vi "__RunTestsInCurrentProject.vi"() -> ()   [LabVIEW 2019]
uses:
  TestResult/TestResult.lvclass
  TestRunner/TestRunner.lvclass
  <vilib>/Analysis/baseanly.llb/Mean (DBL).vi
  TestSuite/TestSuite.lvclass
  TestFailure/TestFailure.lvclass
  CodeCoverage/CodeCoverage.lvclass
  <vilib>/Analysis/NI_AALBase.lvlib
panel:
  out "Not Fully Covered":path[](array[path])
  out "Total Coverage [%]":dbl format="%0.2f"
  out "Time [s]":dbl
  out "Count":i32
  out "error out":errorcluster
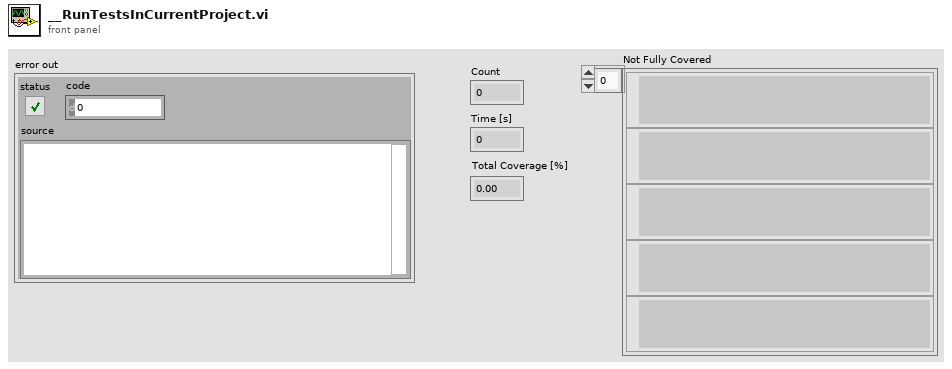
[diagram p1: front panel]
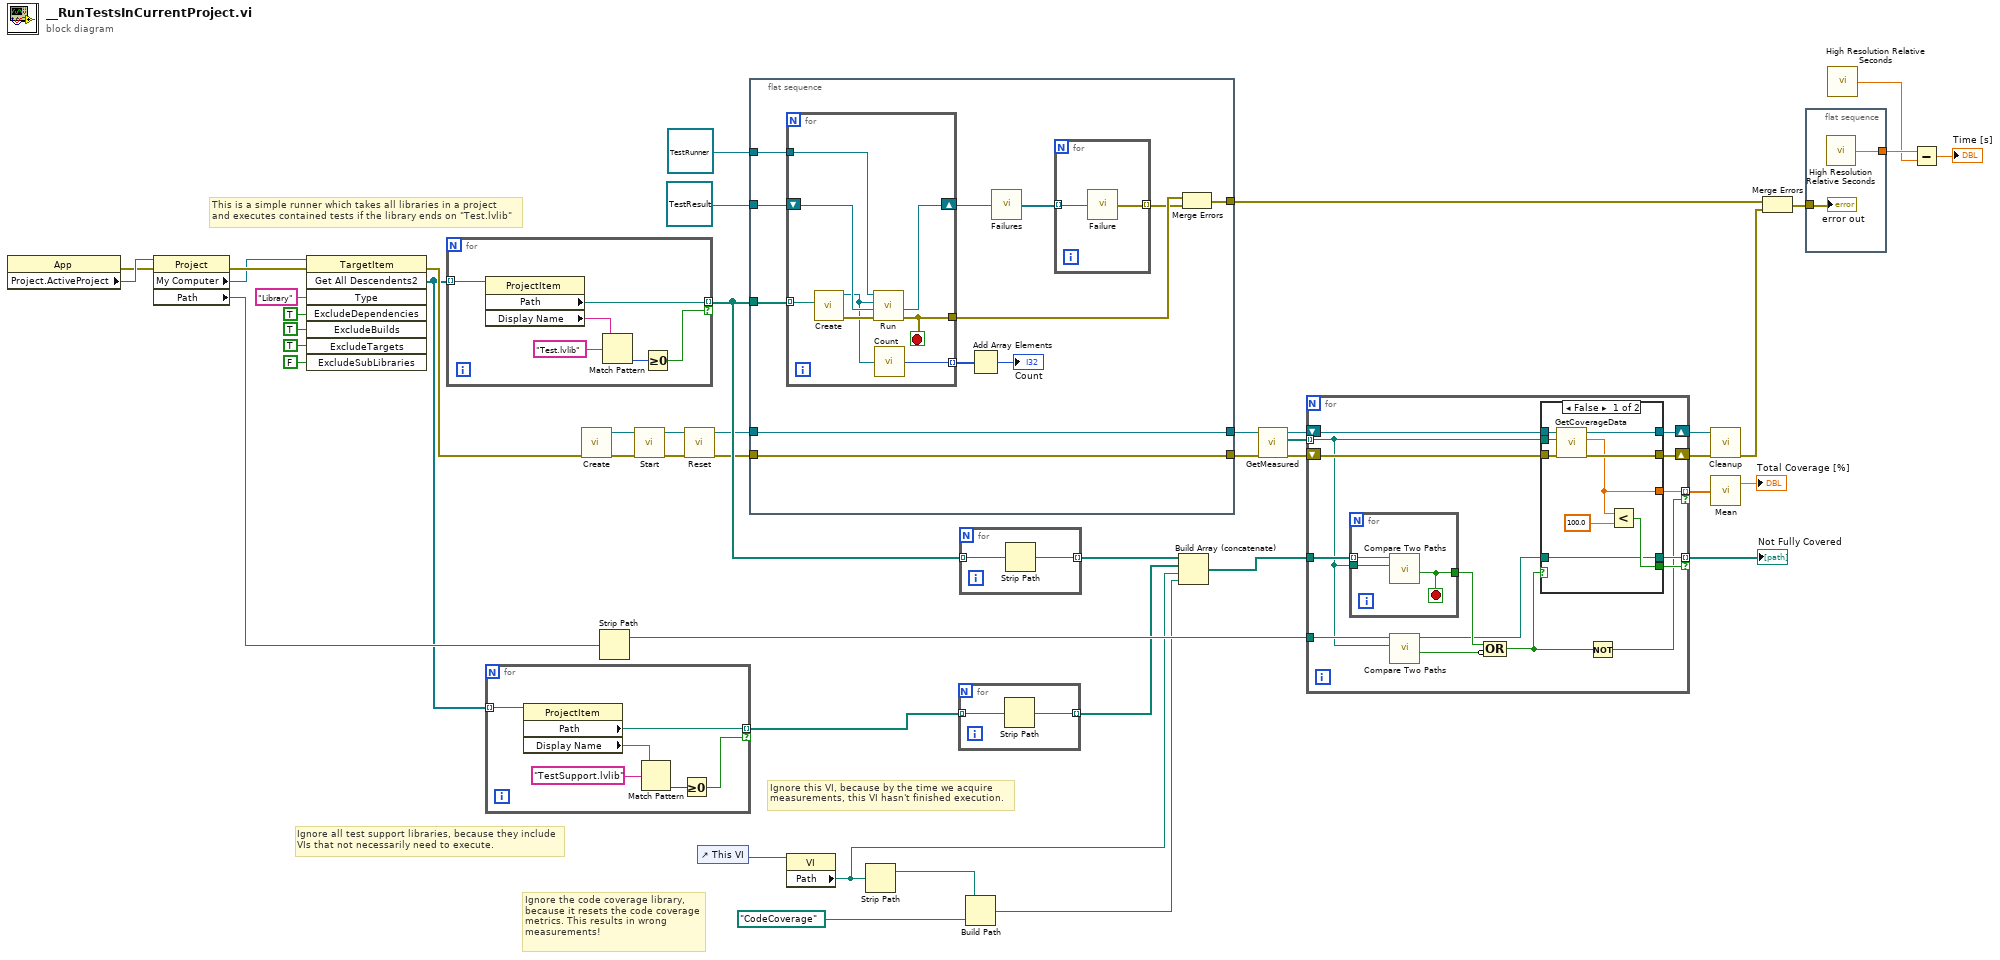
[diagram p0: block diagram]
diagram:
  # "Ignore all test support libraries, because they include\nVIs that not necessarily need to execute."
  # "Ignore this VI, because by the time we acquire\nmeasurements, this VI hasn't finished execution."
  # "Ignore the code coverage library,\nbecause it resets the code coverage\nmetrics. This results in wrong\nmeasurements!"
  # "This is a simple runner which takes all libraries in a project\nand executes contained tests if the library ends on \"Test.lvlib\""
  n1 = property class="App"() -> (error out=w46:errorcluster, "Project.ActiveProject"=w47:refnum<vi>)  [unwired: 2 in, 1 out]
  n2 = property class="Project"(reference=w47, error in=w46) -> (error out=w45:errorcluster, "My Computer"=w34:refnum<vi>, "Path"=w18:path)  [unwired: 1 out]
  n3 = invoke class="TargetItem" method="Get All Descendents2"(reference=w34, error in=w45, "Type"="Library", "ExcludeDependencies"=TRUE, "ExcludeBuilds"=TRUE, "ExcludeTargets"=TRUE, "ExcludeSubLibraries"=FALSE) -> (error out=w20:errorcluster, "Get All Descendents2"=w14:refnum<vi>[])  [unwired: 1 in, 6 out]
  n4 = for {
    tunnel: w14 -> [w53] mode=indexing
    tunnel: [w49] -> w17 mode=indexing if=w48
    n5 = property class="ProjectItem"(reference=w53) -> ("Path"=w49:path, "Display Name"=w50:string)  [unwired: 1 in, 2 out]
    n6 = Match Pattern(string=w50, regular expression="Test.lvlib") -> (offset past match=w51:i32)  [unwired: 1 in, 3 out]
    n7 = Greater Or Equal To 0?(x=w51) -> (x >= 0?=w48:bool)
  }
  n8 = for {
    tunnel: w14 -> [w59] mode=indexing
    tunnel: [w55] -> w13 mode=indexing if=w54
    n9 = property class="ProjectItem"(reference=w59) -> ("Path"=w55:path, "Display Name"=w56:string)  [unwired: 1 in, 2 out]
    n10 = Match Pattern(string=w56, regular expression="TestSupport.lvlib") -> (offset past match=w57:i32)  [unwired: 1 in, 3 out]
    n11 = Greater Or Equal To 0?(x=w57) -> (x >= 0?=w54:bool)
  }
  n12 = call "Create.vi"("error in (no error)"=w20) -> ("error out"=w31:errorcluster, "CodeCoverage out"=w4:refnum<class "CodeCoverage.lvclass">)  [unwired: 9 in]
  n13 = Strip Path(path=w18) -> (stripped path=w15:path)  [unwired: 1 out]
  n14 = call "Start.vi"("error in (no error)"=w31, "CodeCoverage in"=w4) -> ("error out"=w6:errorcluster, "CodeCoverage out"=w3:refnum<class "CodeCoverage.lvclass">)  [unwired: 8 in]
  n15 = call "Reset.vi"("error in (no error)"=w6, "CodeCoverage in"=w3) -> ("error out"=w5:errorcluster, "CodeCoverage out"=w2:refnum<class "CodeCoverage.lvclass">)  [unwired: 8 in]
  n16 = control-ref of="This VI"() -> (w10:refnum<vi>)
  n17 = flat-sequence {
    tunnel: w17 -> [w71]
    tunnel: refnum<class "TestResult.lvclass"> refnum ("TestResult out") -> [w70]
    tunnel: [w65] -> w29
    tunnel: refnum<class "TestRunner.lvclass"> refnum ("TestRunner in") -> [w64]
    tunnel: [w61] -> w23
    tunnel: w2 -> [w61]
    tunnel: [w60] -> w32
    tunnel: w5 -> [w60]
    frame #0 {
      n18 = for {
        tunnel: w71 -> [w81] mode=indexing
        shift-right: [w79] -> w69
        shift-left: w70 -> [w80]
        tunnel: [w77] -> w67
        tunnel: w64 -> [w76]
        tunnel: [w74] -> w63 mode=indexing
        stop <- w77 stop-if-true
        n19 = call "Create.vi"("Path"=w81) -> ("error out"=w78:errorcluster, "TestSuite"=w75:refnum<class "TestSuite.lvclass">)  [unwired: 9 in]
        n20 = call-dynamic "Run.vi"("error in (no error)"=w78, "TestResult"=w80, "TestSuite"=w75, "TestRunner in"=w76) -> ("error out"=w77:errorcluster, "TestResult out"=w79:refnum<class "TestResult.lvclass">)  [unwired: 5 in, 1 out]
        n21 = call "Count.vi"("TestSuite In"=w75) -> ("Count"=w74:i32)
      }
      n22 = Add Array Elements(numeric array=w63) -> (sum=→"Count":i32)
      n23 = call "Failures.vi"("TestResult In"=w69) -> ("Failures"=w68:refnum<class "TestFailure.lvclass">[])
      n24 = for {
        tunnel: w68 -> [w73] mode=indexing
        tunnel: [w72] -> w66 mode=indexing
        n25 = call "Failure.vi"("TestFailure In"=w73) -> ("Failure"=w72:errorcluster)
      }
      n26 = Merge Errors(w67, w66) -> (w65:errorcluster)
    }
  }
  n27 = property class="VI"(reference=w10) -> ("Path"=w7:path)  [unwired: 1 in, 2 out]
  n28 = Strip Path(path=w7) -> (stripped path=w8:path)  [unwired: 1 out]
  n29 = for {
    tunnel: w13 -> [w83] mode=indexing
    tunnel: [w82] -> w11 mode=indexing
    n30 = Strip Path(path=w83) -> (stripped path=w82:path)  [unwired: 1 out]
  }
  n31 = for {
    tunnel: w17 -> [w85] mode=indexing
    tunnel: [w84] -> w16 mode=indexing
    n32 = Strip Path(path=w85) -> (stripped path=w84:path)  [unwired: 1 out]
  }
  n33 = Build Path(base path=w8, name or relative path=path "CodeCoverage") -> (appended path=w1:path)
  n34 = Build Array (concatenate)(w16, w11, w7, w1) -> (w12:path[])
  n35 = call "GetMeasured.vi"("error in (no error)"=w32, "CodeCoverage in"=w23) -> ("error out"=w24:errorcluster, "All VIs Measured"=w21:path[], "CodeCoverage out"=w22:refnum<class "CodeCoverage.lvclass">)  [unwired: 7 in]
  n36 = for {
    shift-right: [w99] -> w33
    shift-left: w22 -> [w100]
    shift-right: [w97] -> w30
    shift-left: w24 -> [w98]
    tunnel: [w96] -> w26 mode=indexing if=w87
    tunnel: w21 -> [w91] mode=indexing
    tunnel: [w93] -> w19 mode=indexing if=w95
    tunnel: w12 -> [w94]
    tunnel: w15 -> [w92]
    n37 = for {
      tunnel: [w101] -> w90
      tunnel: w91 -> [w102]
      tunnel: w94 -> [w103] mode=indexing
      stop <- w101 stop-if-true
      n38 = call <vilib>:"Compare Two Paths.vi"("Path 2"=w102, "Path 1"=w103) -> ("Path 2 Relative to Path 1?"=w101:bool)  [unwired: 6 in, 3 out]
    }
    n39 = call <vilib>:"Compare Two Paths.vi"("Path 2"=w91, "Path 1"=w92) -> ("Path 2 Relative to Path 1?"=w89:bool, "Relative Path from 1 to 2"=w86:path)  [unwired: 6 in, 2 out]
    n40 = Compound Arithmetic op=OR(w90, invert w89) -> (w88:bool)
    n41 = case shown="False" w88 {
      tunnel: w100 -> [w112 w113]
      tunnel: [w111 w113] -> w99
      tunnel: w98 -> [w110 w114]
      tunnel: [w109 w114] -> w97
      tunnel: [w108 _] -> w96
      tunnel: [w106 _] -> w95
      tunnel: w91 -> [w105 _]
      tunnel: [w104 _] -> w93
      tunnel: w86 -> [w104 _]
      frame False {
        n42 = call "GetCoverageData.vi"("error in (no error)"=w110, "VI Path"=w105, "CodeCoverage in"=w112) -> ("error out"=w109:errorcluster, "Coverage Percentage"=w108:dbl, "CodeCoverage out"=w111:refnum<class "CodeCoverage.lvclass">)  [unwired: 6 in]
        n43 = Less?(x=w108, y=100.0) -> (x < y?=w106:bool)
      }
      frame True {
      }
    }
    n44 = Not(x=w88) -> (.not. x?=w87:bool)
  }
  "Not Fully Covered" <- w19
  n45 = call "Cleanup.vi"("error in (no error)"=w30, "CodeCoverage in"=w33) -> ("error out"=w27:errorcluster)  [unwired: 9 in]
  n46 = call-poly <vilib>:"Mean.vi"("X"=w26) -> ("mean"=→"Total Coverage [%]":dbl)  [unwired: 1 out]
  n47 = Merge Errors(w29, w27) -> (w28:errorcluster)
  n48 = flat-sequence {
    tunnel: w28 -> [w116]
    tunnel: [w115] -> w37
    frame #0 {
      n49 = call <vilib>:"High Resolution Relative Seconds.vi"() -> ("relative seconds"=w115:dbl)
      "error out" <- w116
    }
  }
  n50 = call <vilib>:"High Resolution Relative Seconds.vi"() -> ("relative seconds"=w36:dbl)
  n51 = Subtract(x=w37, y=w36) -> (x-y=→"Time [s]":dbl)
